vi "GetLVDirectoryPath.vi"() -> (0 "error out":errorcluster, 3 "LV Path":string)   [LabVIEW 2010, in "CustomProjectLibrary.lvlib"]
uses:
  CustomProjectLibrary.lvlib
  <vilib>/registry/registry.llb/Registry RtKey.ctl
  <vilib>/registry/registry.llb/Read Registry Value Simple STR.vi
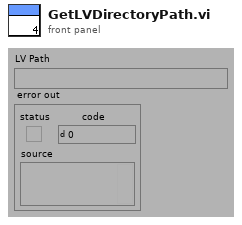
[diagram p1: front panel]
types:
  T1 = typedef "Registry RtKey.ctl" = enum32{"HKEY_CLASSES_ROOT", "HKEY_CURRENT_USER", "HKEY_LOCAL_MACHINE", "HKEY_USERS", "HKEY_PERFORMANCE_DATA", "HKEY_CURRENT_CONFIG", "HKEY_DYN_DATA"}
  T2 = typedef "Registry refnum.ctl" = refnum<k1>
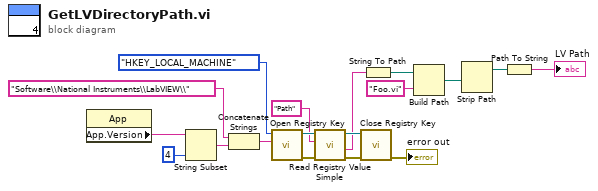
[diagram p0: block diagram]
diagram:
  n1 = property class="App"() -> ("App.Version"=w11:string)  [unwired: 2 in, 2 out]
  n2 = String Subset(string=w11, length (rest)=4 ("length (rest)")) -> (substring=w8:string)  [unwired: 1 out]
  n3 = Concatenate Strings("Software\\National Instruments\\LabVIEW\\" ("subkey"), w8) -> (w7:string)
  n4 = call <vilib>:"Open Registry Key.vi"("subkey"=w7, "root key (HKEY_LOCAL_MACHINE)"=Registry_RtKey."HKEY_LOCAL_MACHINE") -> ("error out"=w17:errorcluster, "refnum out"=w18:T2)  [unwired: 1 in, 7 out]
  n5 = call-poly <vilib>:"Read Registry Value Simple.vi"("error in (no error)"=w17, "value"="Path", "refnum"=w18) -> ("error out"=w15:errorcluster, "String/Binary data"=w6:string, "refnum out"=w14:T2)  [unwired: 1 in, 3 out]
  n6 = call <vilib>:"Close Registry Key.vi"("error in (no error)"=w15, "refnum"=w14) -> ("error out"=→"error out":errorcluster)  [unwired: 5 out]
  n7 = String To Path(string=w6) -> (path=w5:path)
  n8 = Build Path(base path=w5, name or relative path="Foo.vi") -> (appended path=w3:path)
  n9 = Strip Path(path=w3) -> (stripped path=w2:path)  [unwired: 1 out]
  n10 = Path To String(path=w2) -> (string=→"LV Path":string)
